vi "main_Agilent.vi"() -> ()   [LabVIEW 2017]
doc: "Эта версия для работы с системой сбора данных Agilent 34980A"
uses:
  <vilib>/Utility/file.llb/Write Delimited Spreadsheet (string).vi
panel:
  in  "8 or 16":u16(ring)=1 items=["8 chip", "16 chip"]
  in  "Speed record":u16(ring)=1 items=["Fast", "Slow"]
  out "Volt_2":dbl caption="V_2"
  out "Volt_1":dbl caption="V_1"
  out "Fast array":dbl[][](array[numeric])
  in  "Emulate":bool
  out "Boolean":bool
  out "Slow array":string[][](array[string])
  out "timer, s":dbl
  out "ArrayTime":dbl[](array[numeric])
  out "Waveform Graph":dbl[][](graph)
  in  "Wait, sec":u32
  in  "Record Data":bool
  out "error out":errorcluster
  in  "Save Button":bool
  # "s."
  # "В"
  # "В"
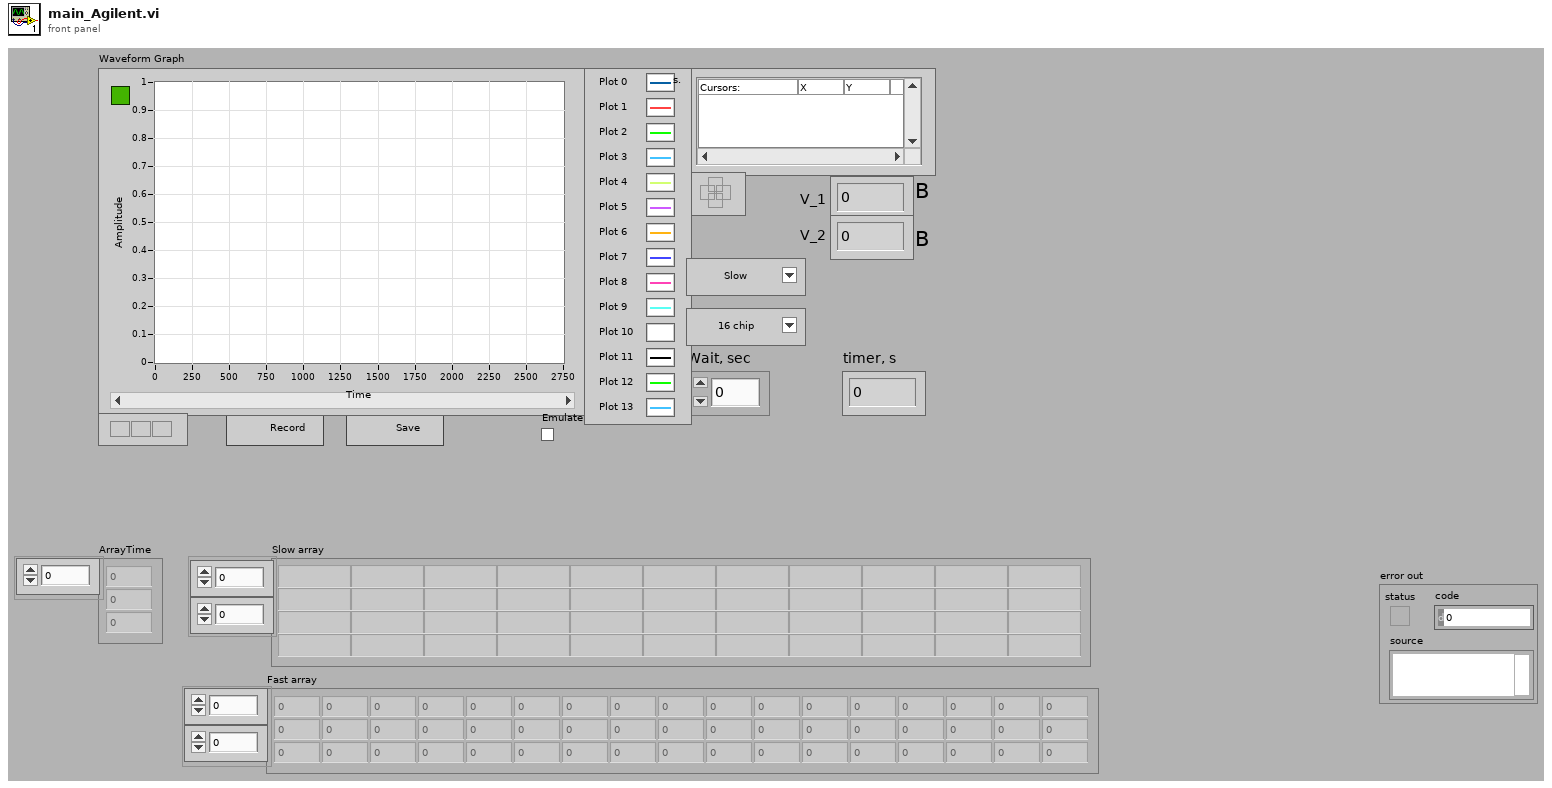
[diagram p1: front panel]
types:
  T1 = cluster{"Microchip_1":dbl[], "Microchip_2":dbl[], "Microchip_3":dbl[], "Microchip_4":dbl[], "Microchip_5":dbl[], "Microchip_6":dbl[], "Microchip_7":dbl[], "Microchip_8":dbl[], "Microchip_9":dbl[], "Microchip_10":dbl[], "Microchip_11":dbl[], "Microchip_12":dbl[], "Microchip_13":dbl[], "Microchip_14":dbl[], "Volt_1":dbl[], "Volt_2":dbl[]}
  T2 = enum8{"Enabled", "Disabled", "Disabled and Grayed Out"}
  T3 = cluster{"Commutator34980A":refnum<visa-resource-name>, "Multimetr34410A":refnum<visa-resource-name>}
  T4 = cluster{"Microchip_1":string[], "Microchip_2":string[], "Microchip_3":string[], "Microchip_4":string[], "Microchip_5":string[], "Microchip_6":string[], "Microchip_7":string[], "Microchip_8":string[], "Microchip_9":string[], "Microchip_10":string[], "Microchip_11":string[], "Microchip_12":string[], "Microchip_13":string[], "Microchip_14":string[], "Volt_1":string[], "Volt_2":string[]}
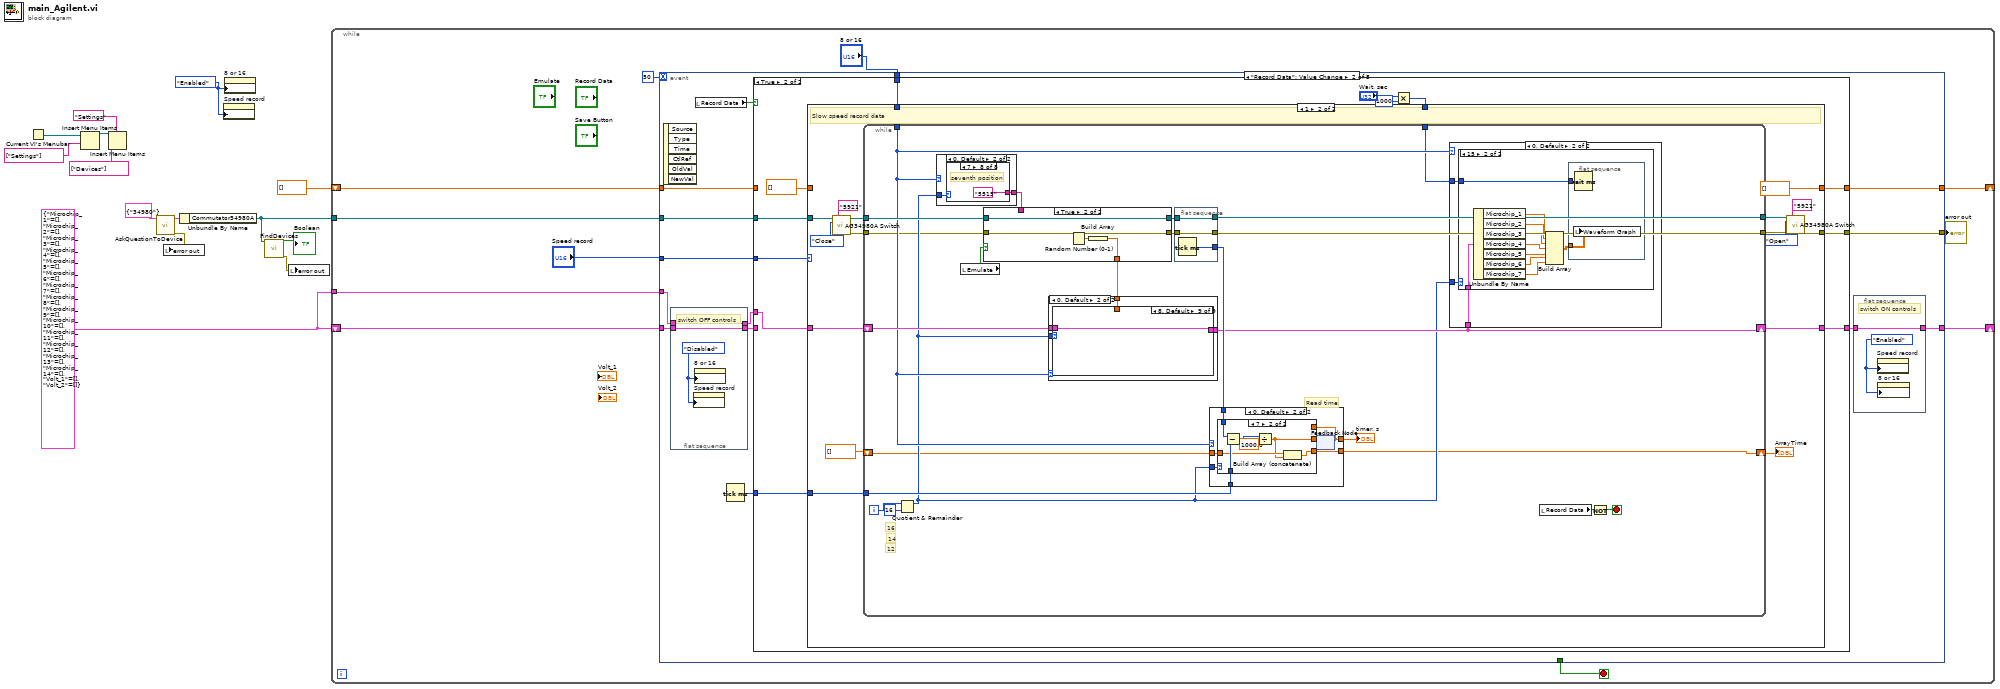
[diagram p0: block diagram]
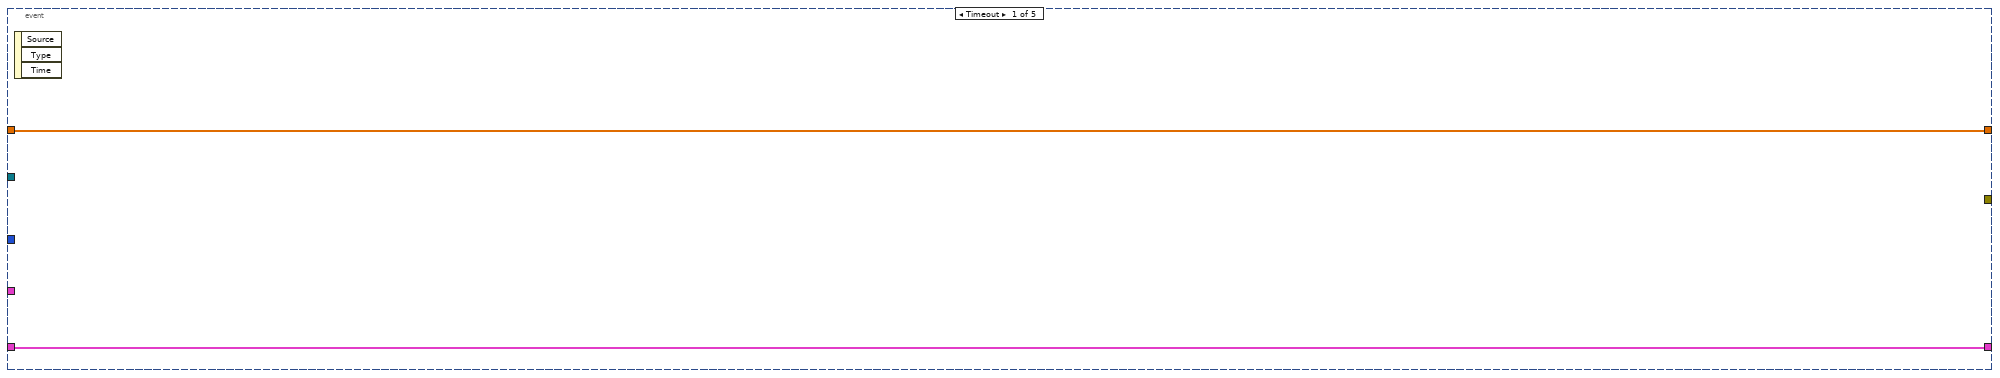
[diagram p2: hidden frame]
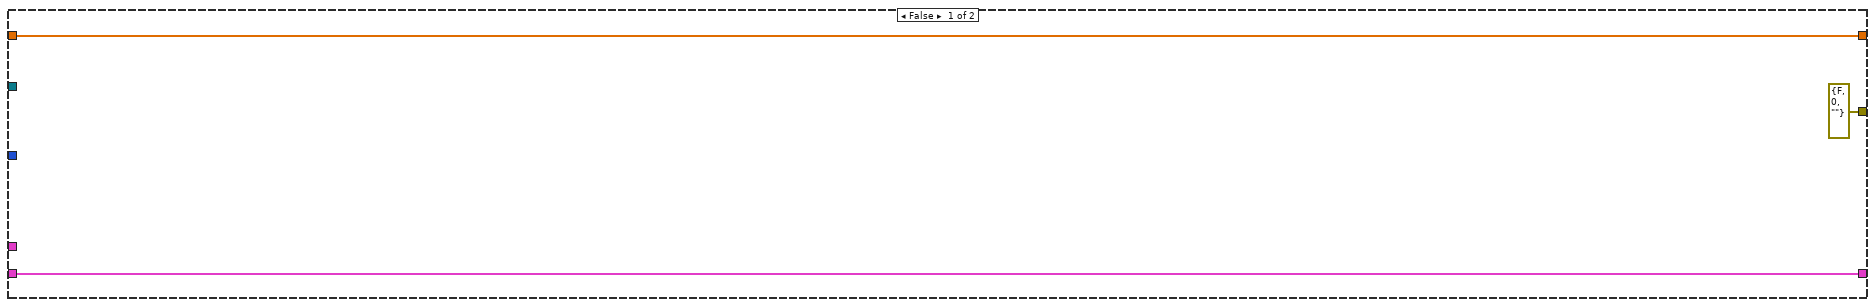
[diagram p3: hidden frame]
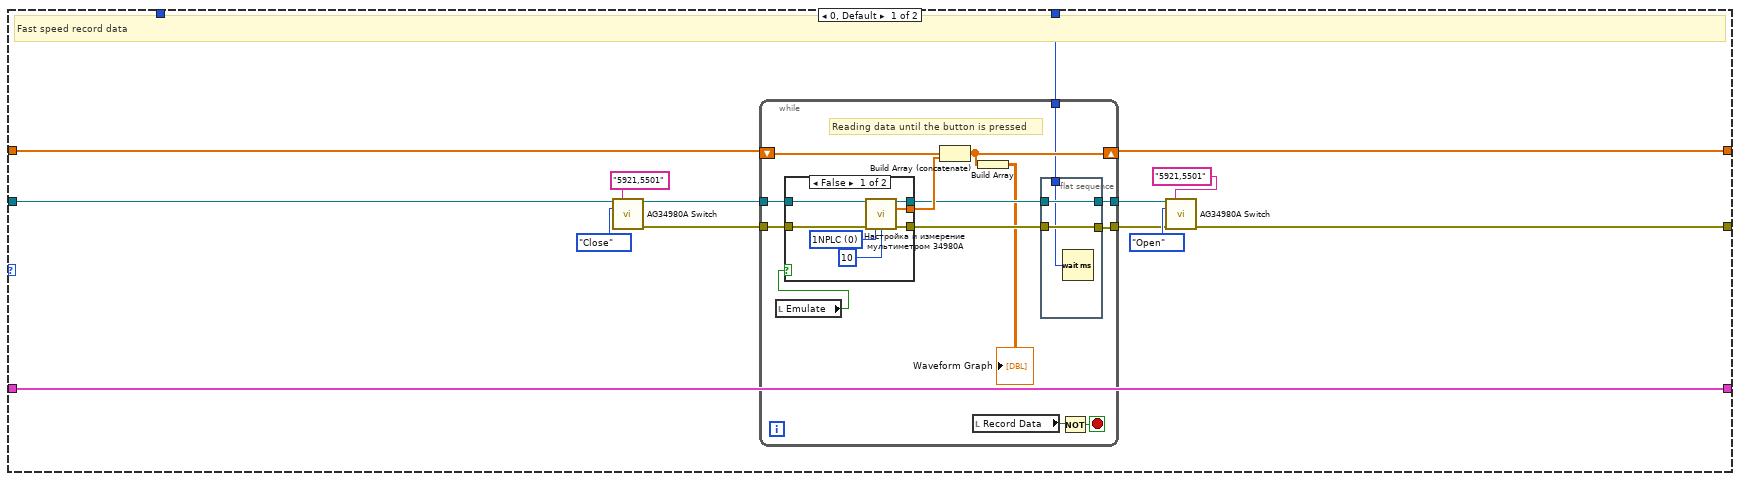
[diagram p4: hidden frame]
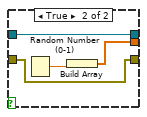
[diagram p5: hidden frame]
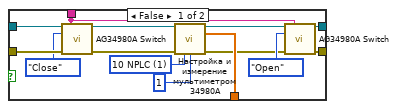
[diagram p6: hidden frame]
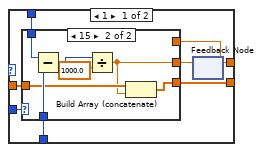
[diagram p7: hidden frame]
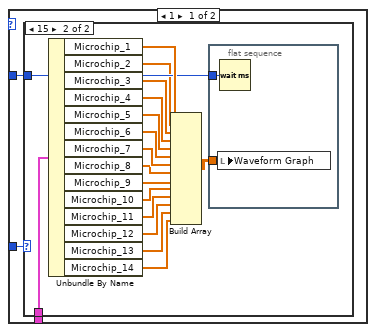
[diagram p10: hidden frame]
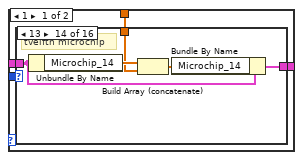
[diagram p13: hidden frame]
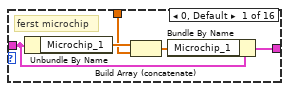
[diagram p14: hidden frame]
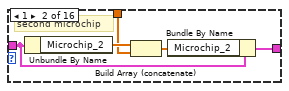
[diagram p15: hidden frame]
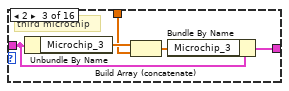
[diagram p16: hidden frame]
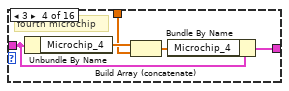
[diagram p17: hidden frame]
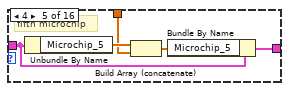
[diagram p18: hidden frame]
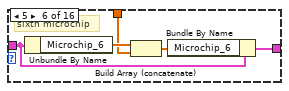
[diagram p19: hidden frame]
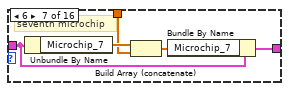
[diagram p20: hidden frame]
diagram:
  w5 = T1 {"Microchip_1"=[], "Microchip_2"=[], "Microchip_3"=[], "Microchip_4"=[], "Microchip_5"=[], "Microchip_6"=[], "Microchip_7"=[], "Microchip_8"=[], "Microchip_9"=[], "Microchip_10"=[], "Microchip_11"=[], "Microchip_12"=[], "Microchip_13"=[], "Microchip_14"=[], "Volt_1"=[], "Volt_2"=[]} ("Cluster Microchip")
  w1 = T2."Enabled" ("Disabled")
  n1 = Current VI's Menubar() -> (w12:refnum<k9>)
  n2 = Insert Menu Items(7:string[] ["Settings"] ("item tags"), 9:w12) -> (3:w11:refnum<k9>)  [unwired: 4 in, 2 out]
  n3 = Insert Menu Items(5:"Settings" ("menu tag"), 7:string[] ["Devices"] ("item tags"), 9:w11) -> ()  [unwired: 3 in, 3 out]
  n4 = call "AskQuestionToDevice .vi"("ClusterNameDevices"=cluster{"Commutator34980A":string} {"Commutator34980A"="34980"}) -> ("error out"=w6:errorcluster, "ClusterAdresDevices"=w7:T3)  [unwired: 9 in]
  n5 = local write "error out"(w6) -> ()
  n6 = Unbundle By Name(w7) -> ("Commutator34980A"=w2:refnum<visa-resource-name>)
  n7 = property on="Speed record" class="Ring (strict)"("DisabledEnum"=w1) -> ()  [unwired: 2 in, 2 out]
  n8 = property on="8 or 16" class="Ring (strict)"("DisabledEnum"=w1) -> ()  [unwired: 2 in, 2 out]
  n9 = call "FindDevices.vi"("Коммутатор Agilent 34980A"=w2) -> ("Статус коммутатора"=→"Boolean":bool, "error out"=w4:errorcluster)  [unwired: 10 in, 3 out]
  n10 = local write "error out"(w4) -> ()
  n11 = while {
    shift-right: [w22] -> _
    shift-left: dbl[] [] -> [w23]
    shift-right: [w20] -> _
    shift-left: w5 -> [w18]
    tunnel: w2 -> [w19]
    tunnel: w5 -> [w17]
    stop <- w24 stop-if-true
    n12 = event shown="[1] \"Record Data\": Value Change" {
      selector: _ -> [_ _ _ _ _]
      dyn-events: _ -> [_ _ _ _ _]
      timeout: 50 -> [_ _ _ _ _]
      tunnel: [_ _ _ _ TRUE] -> w24
      tunnel: w23 -> [w26 w35 w400 _ _]
      tunnel: [w26 w41 _ _ _] -> w22
      tunnel: w19 -> [_ w40 _ _ _]
      tunnel: [_ w39 _ _ _] -> w21
      tunnel: w18 -> [w27 w32 w397 w447 w448]
      tunnel: [w27 w33 _ w447 w448] -> w20
      tunnel: "Speed record" -> [_ w37 w399 _ _]
      tunnel: "8 or 16" -> [_ w36 w395 _ _]
      tunnel: w17 -> [_ w29 _ _ _]
      event Timeout {
        n13 = event-data() -> ()  [unwired: 1 in, 3 out]
      }
      event "Record Data": Value Change {
        n14 = event-data() -> ()  [unwired: 1 in, 6 out]
        n15 = flat-sequence {
          tunnel: w32 -> [w44]
          tunnel: [w44] -> w31
          tunnel: w29 -> [w43]
          tunnel: [w43] -> w28
          frame #0 {
            w42 = T2."Disabled" ("Disabled")
            # "switch OFF controls"
            n16 = property on="Speed record" class="Ring (strict)"("DisabledEnum"=w42) -> ()  [unwired: 2 in, 2 out]
            n17 = property on="8 or 16" class="Ring (strict)"("DisabledEnum"=w42) -> ()  [unwired: 2 in, 2 out]
          }
        }
        n18 = local read "Record Data"() -> (w30:bool)
        n19 = Tick Count (ms)() -> (millisecond timer value=w38:u32)
        n20 = case shown="True" w30 {
          tunnel: w35 -> [w49 _]
          tunnel: [w49 w61] -> w41
          tunnel: w40 -> [_ w60]
          tunnel: [errorcluster {"status"=FALSE, "code"=0, "source"=""} ("error out") w59] -> w39
          tunnel: w31 -> [w48 _]
          tunnel: [w48 w58] -> w34
          tunnel: w38 -> [_ w57]
          tunnel: w37 -> [_ w56]
          tunnel: w36 -> [_ w55]
          tunnel: w28 -> [_ w50]
          frame False {
          }
          frame True {
            n21 = Multiply(x="Wait, sec", y=u32 1000) -> (x*y=w52:u32)
            n22 = case shown="1" w56 {
              tunnel: dbl[] [] -> [w75 _]
              tunnel: [w74 dbl[] []] -> w61
              tunnel: w60 -> [w73 w115]
              tunnel: [w67 w109] -> w59
              tunnel: w50 -> [w63 w120]
              tunnel: [w63 w119] -> w58
              tunnel: w52 -> [w62 w118]
              tunnel: w57 -> [_ w117]
              tunnel: w55 -> [_ w107]
              frame 0, Default {
                # "Fast speed record data"
                n23 = call "AG34980A Switch.vi"("VISA resource name"=w73, "Channel List"="5921,5501", "Open/Close (0:Close)"=enum16{"Close", "Open"}."Close") -> ("VISA resource name out"=w72:refnum<visa-resource-name>, "error out"=w69:errorcluster)  [unwired: 10 in, 1 out]
                n24 = while {
                  shift-right: [w83] -> w74
                  shift-left: w75 -> [w89]
                  tunnel: w72 -> [w85]
                  tunnel: [w80] -> w70
                  tunnel: w69 -> [w84]
                  tunnel: [w78] -> w68
                  tunnel: w62 -> [w77]
                  stop <- w87 stop-if-true
                  # "Reading data until the button is pressed"
                  n25 = local read "Emulate"() -> (w82:bool)
                  n26 = case shown="False" w82 {
                    tunnel: [w99 w101] -> w86
                    tunnel: w85 -> [w98 w103]
                    tunnel: [w97 w103] -> w81
                    tunnel: w84 -> [w96 w100]
                    tunnel: [w95 w100] -> w79
                    frame False {
                      w93 = u16 0 items=["1NPLC", "10 NPLC"] ("Скорост измерения")
                      n27 = call "Настройка и измерение мультиметром 34980A.vi"("Коммутатор Agilent 34980A in"=w98, "error in"=w96, "Скорост измерения"=w93, "Число измерений"=10) -> ("Коммутатор Agilent 34980A out"=w97:refnum<visa-resource-name>, "+U /-U выходное"=w99:dbl[], "error out 2"=w95:errorcluster)  [unwired: 9 in]
                    }
                    frame True {
                      n28 = Random Number (0-1)() -> (number: 0 to 1=w102:dbl)
                      n29 = Build Array(w102) -> (w101:dbl[])
                    }
                  }
                  n30 = Build Array (concatenate)(w89, w86) -> (w83:dbl[])
                  n31 = local read "Record Data"() -> (w88:bool)
                  n32 = Build Array(w83) -> (→"Waveform Graph":dbl[][])
                  n33 = flat-sequence {
                    tunnel: [w92] -> w80
                    tunnel: w81 -> [w92]
                    tunnel: [w91] -> w78
                    tunnel: w79 -> [w91]
                    tunnel: w77 -> [w90]
                    frame #0 {
                      n34 = Wait (ms)(milliseconds to wait=w90) -> ()  [unwired: 1 out]
                    }
                  }
                  n35 = Not(x=w88) -> (.not. x?=w87:bool)
                }
                n36 = call "AG34980A Switch.vi"("VISA resource name"=w70, "Channel List"="5921,5501", "Open/Close (0:Close)"=enum16{"Close", "Open"}."Open", "error in (no error)"=w68) -> ("error out"=w67:errorcluster)  [unwired: 9 in, 2 out]
              }
              frame 1 {
                # "Slow speed record data"
                n37 = call "AG34980A Switch.vi"("VISA resource name"=w115, "Channel List"="5921", "Open/Close (0:Close)"=enum16{"Close", "Open"}."Close") -> ("VISA resource name out"=w114:refnum<visa-resource-name>, "error out"=w104:errorcluster)  [unwired: 10 in, 1 out]
                n38 = while {
                  tunnel: w114 -> [w140]
                  shift-right: [w130] -> w119
                  shift-left: w120 -> [w139]
                  tunnel: w118 -> [w124]
                  tunnel: [w135] -> w108
                  tunnel: w117 -> [w133]
                  tunnel: [w131] -> w110
                  tunnel: w107 -> [w129]
                  shift-right: [w126] -> w105
                  shift-left: dbl[] [] ("ArrayTime 2") -> [w127]
                  tunnel: w104 -> [w123]
                  i -> [w142]
                  stop <- w143 stop-if-true
                  # "16"
                  # "14"
                  # "12"
                  # "Read time"
                  n39 = Quotient & Remainder(x=w142, y=u32 16) -> (x-y*floor(x/y)=w128:u32)  [unwired: 1 out]
                  n40 = case shown="0, Default" w129 {
                    tunnel: w128 -> [w365 w383]
                    tunnel: [w364 w382] -> w137
                    frame 1 {
                      n41 = case shown="15" w365 {
                        tunnel: ["5501" ("Channel List") "5502" ("Channel List") "5503" ("Channel List") "5504" ("Channel List") "5505" ("Channel List") "5506" ("Channel List") "5507" ("Channel List") "5508" ("Channel List") "5509" ("Channel List") "5510" ("Channel List") "5511" ("Channel List") "5512" ("Channel List") "5513" ("Channel List") "5514" ("Channel List") "5515" ("Channel List") "5516" ("Channel List")] -> w364
                        frame 0, Default {
                          # "ferst position"
                        }
                        frame 1 {
                          # "second position"
                        }
                        frame 2 {
                          # "third position"
                        }
                        frame 3 {
                          # "fourth position"
                        }
                        frame 4 {
                          # "fifth position"
                        }
                        frame 5 {
                          # "sixth position"
                        }
                        frame 6 {
                          # "seventh position"
                        }
                        frame 7 {
                          # "eighth position"
                        }
                        frame 8 {
                          # "ninth position"
                        }
                        frame 9 {
                          # "tenth position"
                        }
                        frame 10 {
                          # "eleventh position"
                        }
                        frame 11 {
                          # "tvelfth position"
                        }
                        frame 12 {
                          # "13 position"
                        }
                        frame 13 {
                          # "14 position"
                        }
                        frame 14 {
                          # "15 position"
                        }
                        frame 15 {
                          # "16 position"
                        }
                      }
                    }
                    frame 0, Default {
                      n42 = case shown="7" w383 {
                        tunnel: ["5501" ("Channel List") "5502" ("Channel List") "5503" ("Channel List") "5504" ("Channel List") "5505" ("Channel List") "5506" ("Channel List") "5507" ("Channel List") "5515" ("Channel List")] -> w382
                        frame 0, Default {
                          # "ferst position"
                        }
                        frame 1 {
                          # "second position"
                        }
                        frame 2 {
                          # "third position"
                        }
                        frame 3 {
                          # "fourth position"
                        }
                        frame 4 {
                          # "fifth position"
                        }
                        frame 5 {
                          # "sixth position"
                        }
                        frame 6 {
                          # "seventh position"
                        }
                        frame 7 {
                          # "seventh position"
                        }
                      }
                    }
                  }
                  n43 = local read "Emulate"() -> (w122:bool)
                  n44 = case shown="True" w122 {
                    tunnel: w140 -> [w158 w159]
                    tunnel: [w157 w161] -> w138
                    tunnel: w137 -> [w156 _]
                    tunnel: [w155 w160] -> w136
                    tunnel: [w154 w159] -> w132
                    tunnel: w123 -> [w153 w160]
                    frame False {
                      w147 = u16 1 items=["1NPLC", "10 NPLC"] ("Скорост измерения")
                      n45 = call "AG34980A Switch.vi"("VISA resource name"=w158, "Channel List"=w156, "Open/Close (0:Close)"=enum16{"Close", "Open"}."Close", "error in (no error)"=w153) -> ("VISA resource name out"=w146:refnum<visa-resource-name>, "error out"=w145:errorcluster)  [unwired: 9 in, 1 out]
                      n46 = call "Настройка и измерение мультиметром 34980A.vi"("Коммутатор Agilent 34980A in"=w146, "error in"=w145, "Скорост измерения"=w147, "Число измерений"=1) -> ("Коммутатор Agilent 34980A out"=w151:refnum<visa-resource-name>, "+U /-U выходное"=w157:dbl[], "error out 2"=w150:errorcluster)  [unwired: 9 in]
                      n47 = call "AG34980A Switch.vi"("VISA resource name"=w151, "Channel List"=w156, "Open/Close (0:Close)"=enum16{"Close", "Open"}."Open", "error in (no error)"=w150) -> ("VISA resource name out"=w154:refnum<visa-resource-name>, "error out"=w155:errorcluster)  [unwired: 9 in, 1 out]
                    }
                    frame True {
                      n48 = Random Number (0-1)() -> (number: 0 to 1=w162:dbl)
                      n49 = Build Array(w162) -> (w161:dbl[])
                    }
                  }
                  n50 = case shown="0, Default" w129 {
                    tunnel: w139 -> [w235 w321]
                    tunnel: w138 -> [w234 w320]
                    tunnel: [w233 w319] -> w130
                    tunnel: w128 -> [w232 w318]
                    frame 1 {
                      n51 = case shown="13" w232 {
                        tunnel: [w236 w241 w246 w251 w256 w261 w266 w271 w276 w281 w286 w291 w296 w301 w308 w314] -> w233
                        tunnel: w235 -> [w237 w242 w247 w252 w257 w262 w267 w272 w277 w282 w287 w292 w297 w302 w309 w315]
                        tunnel: w234 -> [w239 w244 w249 w254 w259 w264 w269 w274 w279 w284 w289 w294 w299 w304 w307 w313]
                        frame 0, Default {
                          # "ferst microchip"
                          n52 = Unbundle By Name(w237) -> ("Microchip_1"=w240:dbl[])
                          n53 = Build Array (concatenate)(w240, w239) -> (w238:dbl[])
                          n54 = Bundle By Name(cluster=w237, "Microchip_1"=w238) -> (w236:T1)
                        }
                        frame 1 {
                          # "second microchip"
                          n55 = Unbundle By Name(w242) -> ("Microchip_2"=w245:dbl[])
                          n56 = Build Array (concatenate)(w245, w244) -> (w243:dbl[])
                          n57 = Bundle By Name(cluster=w242, "Microchip_2"=w243) -> (w241:T1)
                        }
                        frame 2 {
                          # "third microchip"
                          n58 = Unbundle By Name(w247) -> ("Microchip_3"=w250:dbl[])
                          n59 = Build Array (concatenate)(w250, w249) -> (w248:dbl[])
                          n60 = Bundle By Name(cluster=w247, "Microchip_3"=w248) -> (w246:T1)
                        }
                        frame 3 {
                          # "fourth microchip"
                          n61 = Unbundle By Name(w252) -> ("Microchip_4"=w255:dbl[])
                          n62 = Build Array (concatenate)(w255, w254) -> (w253:dbl[])
                          n63 = Bundle By Name(cluster=w252, "Microchip_4"=w253) -> (w251:T1)
                        }
                        frame 4 {
                          # "fifth microchip"
                          n64 = Unbundle By Name(w257) -> ("Microchip_5"=w260:dbl[])
                          n65 = Build Array (concatenate)(w260, w259) -> (w258:dbl[])
                          n66 = Bundle By Name(cluster=w257, "Microchip_5"=w258) -> (w256:T1)
                        }
                        frame 5 {
                          # "sixth microchip"
                          n67 = Unbundle By Name(w262) -> ("Microchip_6"=w265:dbl[])
                          n68 = Build Array (concatenate)(w265, w264) -> (w263:dbl[])
                          n69 = Bundle By Name(cluster=w262, "Microchip_6"=w263) -> (w261:T1)
                        }
                        frame 6 {
                          # "seventh microchip"
                          n70 = Unbundle By Name(w267) -> ("Microchip_7"=w270:dbl[])
                          n71 = Build Array (concatenate)(w270, w269) -> (w268:dbl[])
                          n72 = Bundle By Name(cluster=w267, "Microchip_7"=w268) -> (w266:T1)
                        }
                        frame 7 {
                          # "eighth microchip"
                          n73 = Unbundle By Name(w272) -> ("Microchip_8"=w275:dbl[])
                          n74 = Build Array (concatenate)(w275, w274) -> (w273:dbl[])
                          n75 = Bundle By Name(cluster=w272, "Microchip_8"=w273) -> (w271:T1)
                        }
                        frame 8 {
                          # "ninth microchip"
                          n76 = Unbundle By Name(w277) -> ("Microchip_9"=w280:dbl[])
                          n77 = Build Array (concatenate)(w280, w279) -> (w278:dbl[])
                          n78 = Bundle By Name(cluster=w277, "Microchip_9"=w278) -> (w276:T1)
                        }
                        frame 9 {
                          # "tenth microchip"
                          n79 = Unbundle By Name(w282) -> ("Microchip_10"=w285:dbl[])
                          n80 = Build Array (concatenate)(w285, w284) -> (w283:dbl[])
                          n81 = Bundle By Name(cluster=w282, "Microchip_10"=w283) -> (w281:T1)
                        }
                        frame 10 {
                          # "eleventh microchip"
                          n82 = Unbundle By Name(w287) -> ("Microchip_11"=w290:dbl[])
                          n83 = Build Array (concatenate)(w290, w289) -> (w288:dbl[])
                          n84 = Bundle By Name(cluster=w287, "Microchip_11"=w288) -> (w286:T1)
                        }
                        frame 11 {
                          # "tvelfth microchip"
                          n85 = Unbundle By Name(w292) -> ("Microchip_12"=w295:dbl[])
                          n86 = Build Array (concatenate)(w295, w294) -> (w293:dbl[])
                          n87 = Bundle By Name(cluster=w292, "Microchip_12"=w293) -> (w291:T1)
                        }
                        frame 12 {
                          # "tvelfth microchip"
                          n88 = Unbundle By Name(w297) -> ("Microchip_13"=w300:dbl[])
                          n89 = Build Array (concatenate)(w300, w299) -> (w298:dbl[])
                          n90 = Bundle By Name(cluster=w297, "Microchip_13"=w298) -> (w296:T1)
                        }
                        frame 13 {
                          # "tvelfth microchip"
                          n91 = Unbundle By Name(w302) -> ("Microchip_14"=w305:dbl[])
                          n92 = Build Array (concatenate)(w305, w304) -> (w303:dbl[])
                          n93 = Bundle By Name(cluster=w302, "Microchip_14"=w303) -> (w301:T1)
                        }
                        frame 14 {
                          # "tvelfth microchip"
                          n94 = Unbundle By Name(w309) -> ("Volt_1"=w311:dbl[])
                          n95 = Index Array(array=w307) -> (element=w306:dbl)  [unwired: 1 in]
                          n96 = Build Array (concatenate)(w311, w307) -> (w310:dbl[])
                          n97 = local write "Volt_1"(w306) -> ()
                          n98 = Bundle By Name(cluster=w309, "Volt_1"=w310) -> (w308:T1)
                        }
                        frame 15 {
                          # "tvelfth microchip"
                          n99 = Unbundle By Name(w315) -> ("Volt_2"=w317:dbl[])
                          n100 = Index Array(array=w313) -> (element=w312:dbl)  [unwired: 1 in]
                          n101 = Build Array (concatenate)(w317, w313) -> (w316:dbl[])
                          n102 = local write "Volt_2"(w312) -> ()
                          n103 = Bundle By Name(cluster=w315, "Volt_2"=w316) -> (w314:T1)
                        }
                      }
                    }
                    frame 0, Default {
                      n104 = case shown="8, Default" w318 {
                        tunnel: [w322 w327 w332 w337 w342 w347 w352 w359 w363] -> w319
                        tunnel: w321 -> [w323 w328 w333 w338 w343 w348 w353 w360 w363]
                        tunnel: w320 -> [w325 w330 w335 w340 w345 w350 w355 w358 _]
                        frame 0 {
                          # "ferst microchip"
                          n105 = Unbundle By Name(w323) -> ("Microchip_1"=w326:dbl[])
                          n106 = Build Array (concatenate)(w326, w325) -> (w324:dbl[])
                          n107 = Bundle By Name(cluster=w323, "Microchip_1"=w324) -> (w322:T1)
                        }
                        frame 1 {
                          # "second microchip"
                          n108 = Unbundle By Name(w328) -> ("Microchip_2"=w331:dbl[])
                          n109 = Build Array (concatenate)(w331, w330) -> (w329:dbl[])
                          n110 = Bundle By Name(cluster=w328, "Microchip_2"=w329) -> (w327:T1)
                        }
                        frame 2 {
                          # "third microchip"
                          n111 = Unbundle By Name(w333) -> ("Microchip_3"=w336:dbl[])
                          n112 = Build Array (concatenate)(w336, w335) -> (w334:dbl[])
                          n113 = Bundle By Name(cluster=w333, "Microchip_3"=w334) -> (w332:T1)
                        }
                        frame 3 {
                          # "fourth microchip"
                          n114 = Unbundle By Name(w338) -> ("Microchip_4"=w341:dbl[])
                          n115 = Build Array (concatenate)(w341, w340) -> (w339:dbl[])
                          n116 = Bundle By Name(cluster=w338, "Microchip_4"=w339) -> (w337:T1)
                        }
                        frame 4 {
                          # "fifth microchip"
                          n117 = Unbundle By Name(w343) -> ("Microchip_5"=w346:dbl[])
                          n118 = Build Array (concatenate)(w346, w345) -> (w344:dbl[])
                          n119 = Bundle By Name(cluster=w343, "Microchip_5"=w344) -> (w342:T1)
                        }
                        frame 5 {
                          # "sixth microchip"
                          n120 = Unbundle By Name(w348) -> ("Microchip_6"=w351:dbl[])
                          n121 = Build Array (concatenate)(w351, w350) -> (w349:dbl[])
                          n122 = Bundle By Name(cluster=w348, "Microchip_6"=w349) -> (w347:T1)
                        }
                        frame 6 {
                          # "sixth microchip"
                          n123 = Unbundle By Name(w353) -> ("Microchip_7"=w356:dbl[])
                          n124 = Build Array (concatenate)(w356, w355) -> (w354:dbl[])
                          n125 = Bundle By Name(cluster=w353, "Microchip_7"=w354) -> (w352:T1)
                        }
                        frame 7 {
                          # "sixth microchip"
                          n126 = Unbundle By Name(w360) -> ("Volt_1"=w362:dbl[])
                          n127 = Index Array(array=w358) -> (element=w357:dbl)  [unwired: 1 in]
                          n128 = Build Array (concatenate)(w362, w358) -> (w361:dbl[])
                          n129 = local write "Volt_1"(w357) -> ()
                          n130 = Bundle By Name(cluster=w360, "Volt_1"=w361) -> (w359:T1)
                        }
                        frame 8, Default {
                        }
                      }
                    }
                  }
                  n131 = flat-sequence {
                    tunnel: w136 -> [w394]
                    tunnel: [w394] -> w135
                    tunnel: [w393] -> w134
                    tunnel: w132 -> [w392]
                    tunnel: [w392] -> w131
                    frame #0 {
                      n132 = Tick Count (ms)() -> (millisecond timer value=w393:u32)
                    }
                  }
                  n133 = case shown="0, Default" w129 {
                    tunnel: w134 -> [w169 w185]
                    tunnel: w133 -> [w168 w184]
                    tunnel: [w167 w183] -> w126
                    tunnel: w128 -> [w166 w182]
                    tunnel: w127 -> [w165 w181]
                    tunnel: [w163 w179] -> w125
                    frame 1 {
                      n134 = feedback #1() -> (w163:dbl)  [unwired: 1 in]
                      n135 = case shown="15" w166 {
                        tunnel: w169 -> [_ w178]
                        tunnel: w168 -> [_ w177]
                        tunnel: [w171 w175] -> w167
                        tunnel: w165 -> [w171 w176]
                        tunnel: [w170 w172] -> w164
                        tunnel: w163 -> [w170 _]
                        frame 0, Default {
                        }
                        frame 15 {
                          n136 = Subtract(x=w178, y=w177) -> (x-y=w174:u32)
                          n137 = Divide(x=w174, y=1000.0) -> (x/y=w172:dbl)
                          n138 = Build Array (concatenate)(w176, w172) -> (w175:dbl[])
                        }
                      }
                      n139 = feedback-in #1(w164) -> ()
                    }
                    frame 0, Default {
                      n140 = feedback #2() -> (w179:dbl)  [unwired: 1 in]
                      n141 = case shown="7" w182 {
                        tunnel: w185 -> [_ w194]
                        tunnel: w184 -> [_ w193]
                        tunnel: [w187 w191] -> w183
                        tunnel: w181 -> [w187 w192]
                        tunnel: [w186 w188] -> w180
                        tunnel: w179 -> [w186 _]
                        frame 0, Default {
                        }
                        frame 7 {
                          n142 = Subtract(x=w194, y=w193) -> (x-y=w190:u32)
                          n143 = Divide(x=w190, y=1000.0) -> (x/y=w188:dbl)
                          n144 = Build Array (concatenate)(w192, w188) -> (w191:dbl[])
                        }
                      }
                      n145 = feedback-in #2(w180) -> ()
                    }
                  }
                  "timer, s" <- w125
                  n146 = case shown="0, Default" w129 {
                    tunnel: w130 -> [w197 w219]
                    tunnel: w128 -> [w196 w218]
                    tunnel: w124 -> [w195 w217]
                    frame 1 {
                      n147 = case shown="15" w196 {
                        tunnel: w197 -> [_ w212]
                        tunnel: w195 -> [_ w211]
                        frame 0, Default {
                        }
                        frame 15 {
                          n148 = Unbundle By Name(w212) -> ("Microchip_1"=w214:dbl[], "Microchip_2"=w210:dbl[], "Microchip_3"=w209:dbl[], "Microchip_4"=w208:dbl[], "Microchip_5"=w207:dbl[], "Microchip_6"=w206:dbl[], "Microchip_7"=w205:dbl[], "Microchip_8"=w204:dbl[], "Microchip_9"=w203:dbl[], "Microchip_10"=w202:dbl[], "Microchip_11"=w201:dbl[], "Microchip_12"=w200:dbl[], "Microchip_13"=w199:dbl[], "Microchip_14"=w198:dbl[])
                          n149 = Build Array(w214, w210, w209, w208, w207, w206, w205, w204, w203, w202, w201, w200, w199, w198) -> (w213:dbl[][])
                          n150 = flat-sequence {
                            tunnel: w213 -> [w216]
                            tunnel: w211 -> [w215]
                            frame #0 {
                              n151 = local write "Waveform Graph"(w216) -> ()
                              n152 = Wait (ms)(milliseconds to wait=w215) -> ()  [unwired: 1 out]
                            }
                          }
                        }
                      }
                    }
                    frame 0, Default {
                      n153 = case shown="15" w218 {
                        tunnel: w219 -> [_ w226]
                        tunnel: w217 -> [_ w227]
                        frame 0, Default {
                        }
                        frame 15 {
                          n154 = Unbundle By Name(w226) -> ("Microchip_1"=w229:dbl[], "Microchip_2"=w225:dbl[], "Microchip_3"=w224:dbl[], "Microchip_4"=w223:dbl[], "Microchip_5"=w222:dbl[], "Microchip_6"=w221:dbl[], "Microchip_7"=w220:dbl[])
                          n155 = Build Array(w229, w225, w224, w223, w222, w221, w220) -> (w228:dbl[][])
                          n156 = flat-sequence {
                            tunnel: w228 -> [w231]
                            tunnel: w227 -> [w230]
                            frame #0 {
                              n157 = local write "Waveform Graph"(w231) -> ()
                              n158 = Wait (ms)(milliseconds to wait=w230) -> ()  [unwired: 1 out]
                            }
                          }
                        }
                      }
                    }
                  }
                  n159 = local read "Record Data"() -> (w144:bool)
                  n160 = Not(x=w144) -> (.not. x?=w143:bool)
                }
                "ArrayTime" <- w105
                n161 = call "AG34980A Switch.vi"("VISA resource name"=w110, "Channel List"="5921", "Open/Close (0:Close)"=enum16{"Close", "Open"}."Open", "error in (no error)"=w108) -> ("error out"=w109:errorcluster)  [unwired: 9 in, 2 out]
              }
            }
          }
        }
        n162 = flat-sequence {
          tunnel: w34 -> [w46]
          tunnel: [w46] -> w33
          frame #0 {
            w45 = T2."Enabled" ("Disabled")
            # "switch ON controls"
            n163 = property on="Speed record" class="Ring (strict)"("DisabledEnum"=w45) -> ()  [unwired: 2 in, 2 out]
            n164 = property on="8 or 16" class="Ring (strict)"("DisabledEnum"=w45) -> ()  [unwired: 2 in, 2 out]
          }
        }
      }
      event "Save Button": Value Change {
        n165 = event-data() -> ()  [unwired: 1 in, 6 out]
        n166 = call "PathToRezult.vi"() -> ("pathToRezult"=w396:path)  [unwired: 11 in]
        n167 = call "ReadDecimal.vi"() -> ("Флаг Разделителя"=w398:bool)  [unwired: 11 in]
        n168 = case shown="1" w399 {
          tunnel: w400 -> [w405 _]
          tunnel: w398 -> [w407 w416]
          tunnel: w397 -> [_ w414]
          tunnel: w396 -> [w402 w411]
          tunnel: w395 -> [_ w409]
          frame 0, Default {
            n169 = local read "ArrayTime"() -> (w406:dbl[])
            n170 = Build Array(w406, w405) -> (w404:dbl[][])
            n171 = Transpose 2D Array(2D array=w404) -> (transposed array=w403:dbl[][])
            "Fast array" <- w403
            n172 = Number To Fractional String(use system decimal point (T)=w407, number=w403) -> (F-format string=w401:string[][])  [unwired: 2 in]
            n173 = call-poly <vilib>:"Write Delimited Spreadsheet.vi"("file path (dialog if empty)"=w402, "2D data"=w401) -> ()  [unwired: 12 in, 2 out]
          }
          frame 1 {
            n174 = Number To Fractional String(use system decimal point (T)=w416, number=w414) -> (F-format string=w418:T4)  [unwired: 2 in]
            n175 = case shown="1" w409 {
              tunnel: w418 -> [w436 w446]
              tunnel: [w423 w438] -> w413
              frame 1 {
                n176 = Unbundle By Name(w436) -> ("Microchip_1"=w435:string[], "Microchip_2"=w434:string[], "Microchip_3"=w433:string[], "Microchip_4"=w432:string[], "Microchip_5"=w431:string[], "Microchip_6"=w430:string[], "Microchip_7"=w429:string[], "Microchip_8"=w428:string[], "Microchip_9"=w427:string[], "Microchip_10"=w426:string[], "Microchip_11"=w425:string[], "Microchip_12"=w424:string[], "Microchip_13"=w422:string[], "Microchip_14"=w421:string[], "Volt_1"=w420:string[], "Volt_2"=w419:string[])
                n177 = Build Array (concatenate)(w435, w434, w433, w432, w431, w430, w429, w428, w427, w426, w425, w424, w422, w421, w420, w419) -> (w423:string[])
              }
              frame 0, Default {
                n178 = Unbundle By Name(w446) -> ("Microchip_1"=w445:string[], "Microchip_2"=w444:string[], "Microchip_3"=w443:string[], "Microchip_4"=w442:string[], "Microchip_5"=w441:string[], "Microchip_6"=w440:string[], "Microchip_7"=w439:string[], "Volt_1"=w437:string[])
                n179 = Build Array (concatenate)(w445, w444, w443, w442, w441, w440, w439, w437) -> (w438:string[])
              }
            }
            n180 = local read "ArrayTime"() -> (w417:dbl[])
            n181 = Number To Fractional String(use system decimal point (T)=w416, number=w417) -> (F-format string=w415:string[])  [unwired: 2 in]
            n182 = Build Array (concatenate)(w415) -> (w412:string[])
            n183 = Build Array(w412, w413) -> (w410:string[][])
            n184 = Transpose 2D Array(2D array=w410) -> (transposed array=w408:string[][])
            "Slow array" <- w408
            n185 = call-poly <vilib>:"Write Delimited Spreadsheet.vi"("file path (dialog if empty)"=w411, "2D data"=w408) -> ()  [unwired: 12 in, 2 out]
          }
        }
      }
      event Menu Selection (User) {
        n186 = event-data() -> ()  [unwired: 1 in, 7 out]
      }
      event Application Instance Close; Panel Close {
        n187 = event-data() -> ()  [unwired: 1 in, 3 out]
        n188 = One Button Dialog(message="Кирдык") -> ()  [unwired: 1 in, 1 out]
      }
    }
    "error out" <- w21
  }
